vi "mMc - global.vi"() -> ()   [LabVIEW 2015]
doc: "全局显示控件"
panel:
  out "done":bool
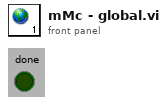
[diagram p1: front panel]
diagram:
